vi "Asylum_Driver_Plugin_IVCurve.vi"(4 "Abort Notifier":refnum<notifier>, 6 "Interpolation":dbl format="%#_13g", 7 "Writing Setpoint":dbl=0.1 format="%#_13g", 8 "error in (no error)":errorcluster, 9 "Offsets":cluster{"X":dbl, "Y":dbl}, 10 "Pattern Data":T2={"Name"="", "Litho"=[], "Set Resistance"=enum."1G ohm", "Meta"=variant}, 11 "Application":refnum<k7>) -> (0 "error out":errorcluster, 1 "Y":dbl[](array[numeric]), 2 "X":dbl[](array[numeric]), 3 "Application Out":refnum<k7>)   [LabVIEW 2019]
uses:
  <userlib>/LevyLab/RemoteControl/RemoteControl/RemoteControl.lvclass
  <userlib>/LevyLab/Instrument Framework/SMOs/RemoteControl/RemoteControl.lvclass
  Classes/Settings/Dot Settings/TypeDefs/IV Settings.ctl
  Classes/Settings/Dot Settings/Dot Settings.lvclass
  <userlib>/LevyLab/RemoteControl/RemoteControl/Typedefs/RC Com Type--enum.ctl
  0e2d323c-3e35-47fb-9129-4c7af1e32b05.vi
  43673bb9-479d-403d-a5d0-439c933431c4.vi
  a6f932bf-8dea-4ae5-a866-4f706d76ef40.vi
  7c826ca2-1f29-4c4d-bf7c-0946160d1343.vi
  0945bc12-bc18-4d8f-896b-f5f56bd4a894.vi
  3a94caf1-4aca-4e02-84db-939cfa50ca80.vi
  <userlib>/LevyLab/Relay Box/Typedefs/Resistor--enum.ctl
  <userlib>/LevyLab/Relay Box/Relay-Box.lvclass
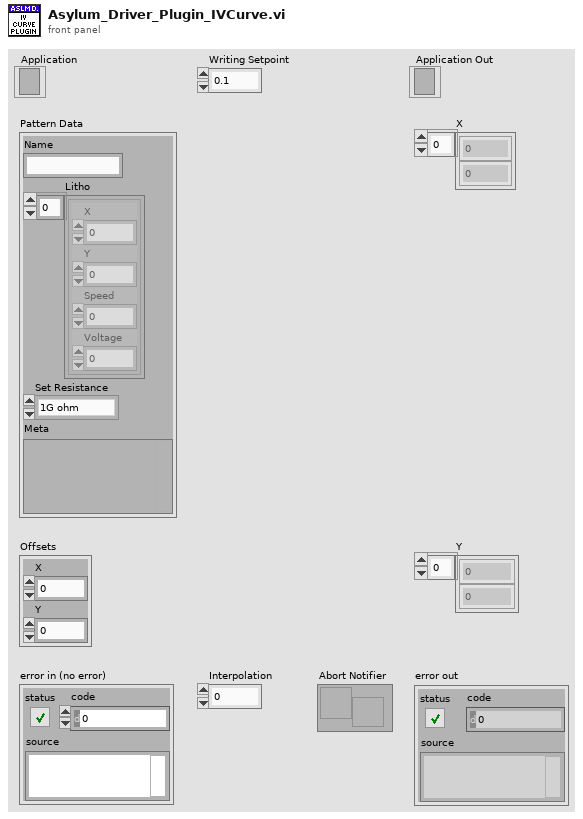
[diagram p1: front panel]
types:
  T1 = typedef "Relay-Box.lvclass/Resistor--enum.ctl" = enum16{"open", "discharge tip", "0 ohms", "100k ohm", "10M ohm", "1G ohm"}
  T2 = cluster{"Name":string, "Litho":cluster{"X":dbl, "Y":dbl, "Speed":dbl, "Voltage":dbl}[], "Set Resistance":T1, "Meta":variant}
  T3 = enum32{"Invalid", "Standard", "Closed", "Hidden", "Minimized", "Maximized"}
  T4 = enum32{"invalid app kind", "Development System", "Run Time System", "Student Edition", "Embedded LabVIEW", "Evaluation", "Custom"}
  T5 = typedef "RemoteControl.lvlib/RemoteControl.lvclass/RC Com Type--enum.ctl" = enum16{"RC", "STM", "ZMQ"}
  T6 = cluster{"Pattern":enum16{"Ramp /", "Ramp /\\", "Smooth Ramp _/", "Smooth Ramp _/\\_", "Frequency"}, "Cycles":i32, "Rate":dbl, "End":dbl, "Start":dbl}
  T7 = enum16{"Ramp /", "Ramp /\\", "Smooth Ramp _/", "Smooth Ramp _/\\_", "Frequency"}
  T8 = typedef "Dot Settings.lvclass/IV Settings.ctl" = cluster{"Pattern":enum16{"Ramp /", "Ramp /\\", "Smooth Ramp _/", "Smooth Ramp _/\\_", "Frequency"}, "Cycles":i32, "Rate":dbl, "End":dbl, "Start":dbl, "Port":u32, "Time":dbl, "Points":dbl[]}
  T9 = cluster{"Core":cluster{"Current VI Reference":refnum<vi>, "Close Panel on Exit?":bool}, "Application":refnum<k7>, "Writing Setpoint":dbl, "Offsets":cluster{"X":dbl, "Y":dbl}, "Interpolation":dbl, "Pattern Data":cluster{"Name":string, "Litho":cluster{"X":dbl, "Y":dbl, "Speed":dbl, "Voltage":dbl}[], "Set Resistance":T1, "Meta":variant}, "Abort Notifier":refnum<notifier>, "RemoteControl":refnum<class "RemoteControl.lvclass">, "IV Settings":T8, "Status":enum16{"IDLE", "RUNNING", "FINISHED", "ABORTED"}, "Timeout":u32, "Plugin Status":i32}
  T10 = cluster{"Current VI Reference":refnum<vi>, "Close Panel on Exit?":bool}
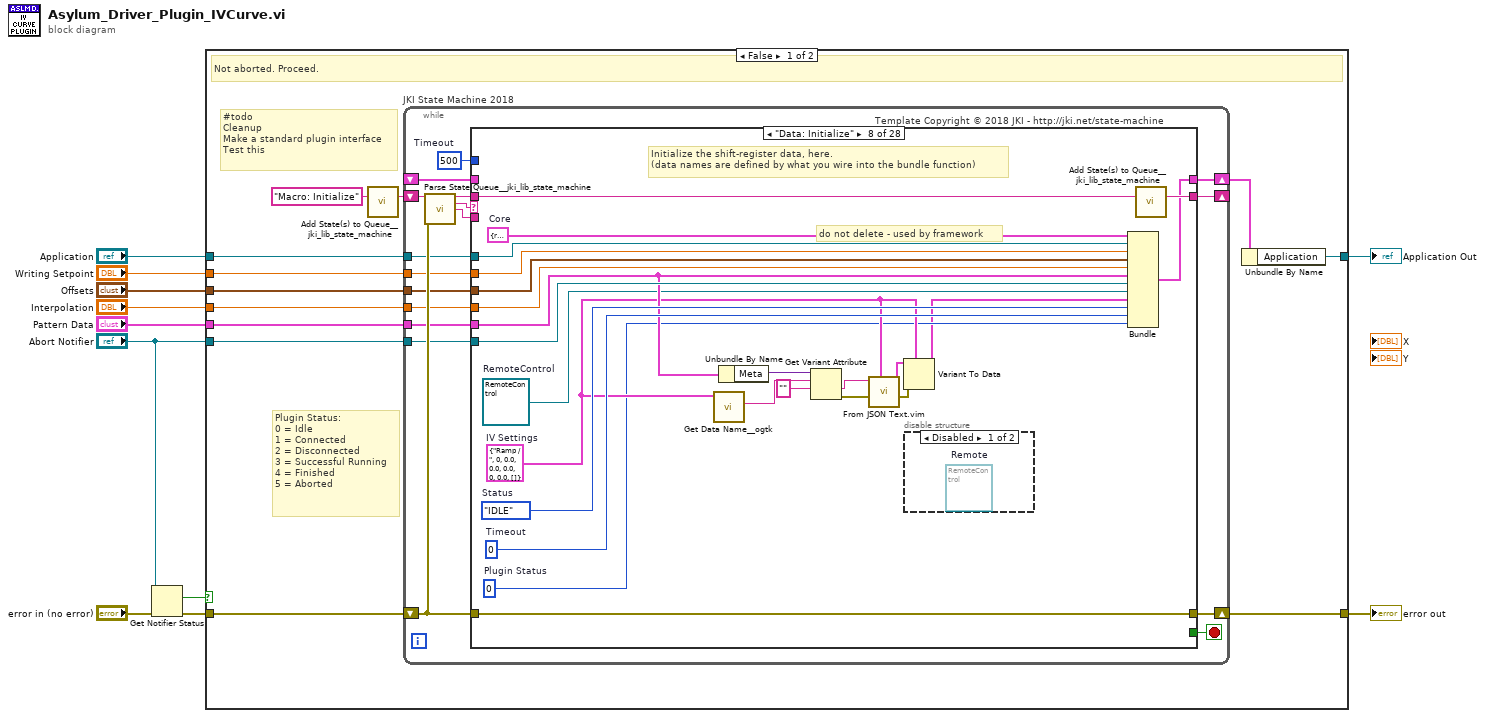
[diagram p0: block diagram]
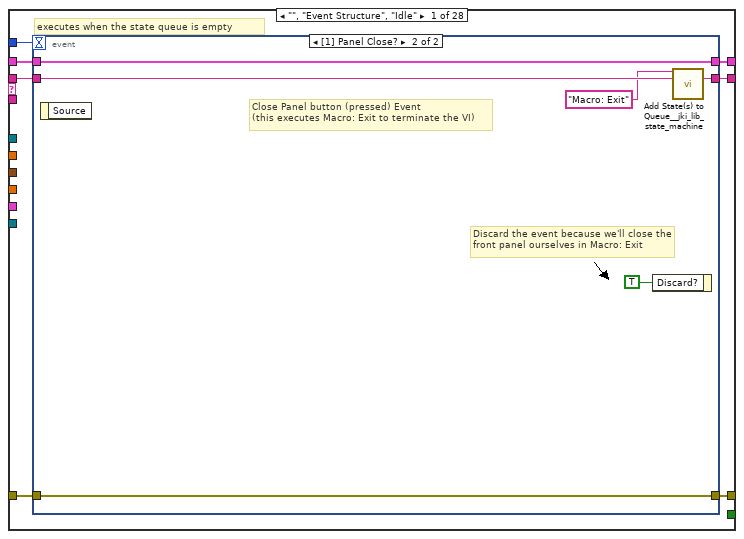
[diagram p2: hidden frame]
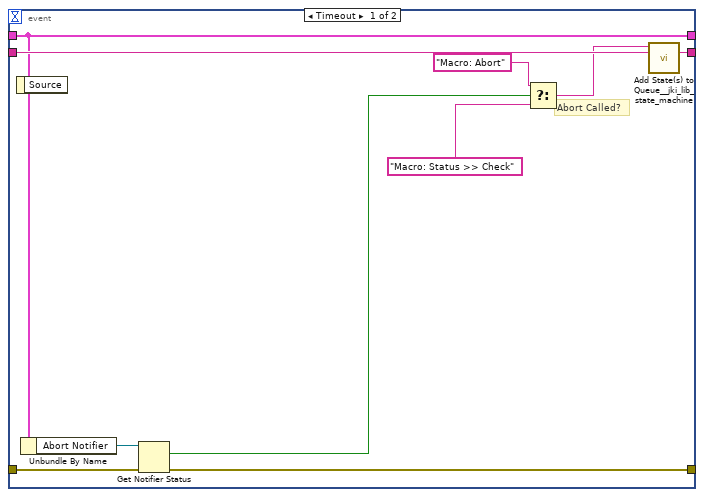
[diagram p3: hidden frame]
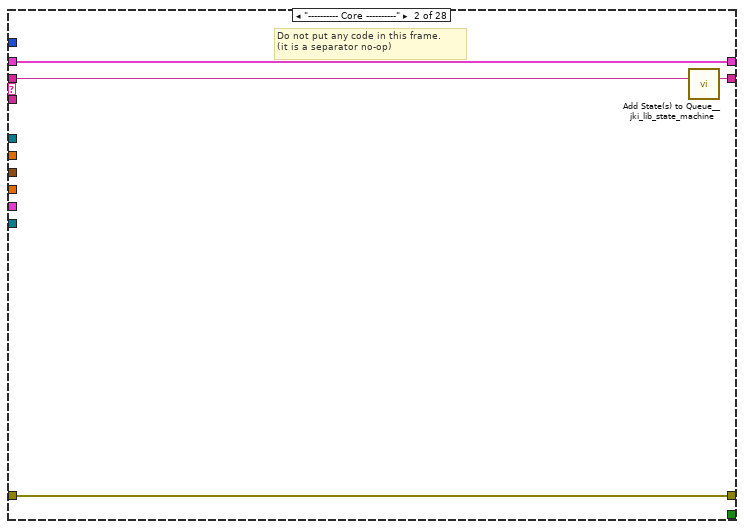
[diagram p4: hidden frame]
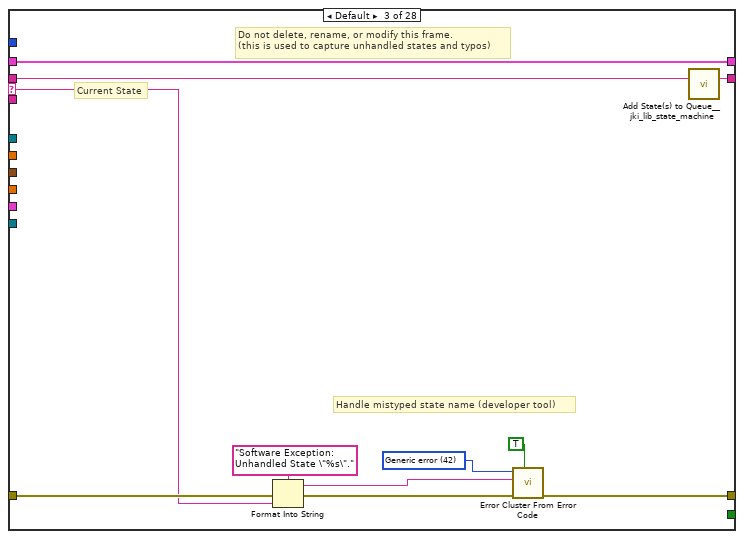
[diagram p5: hidden frame]
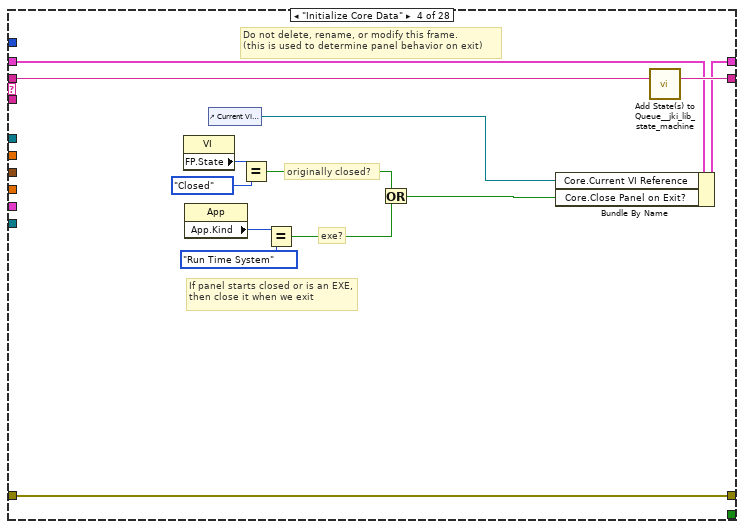
[diagram p6: hidden frame]
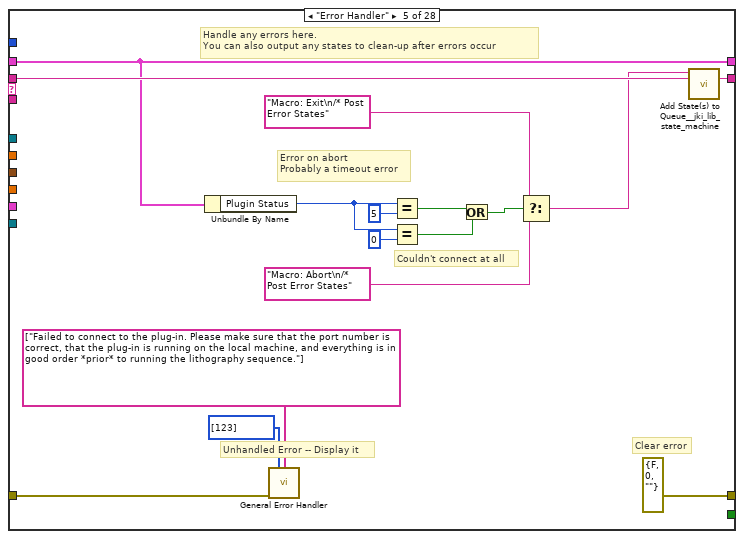
[diagram p7: hidden frame]
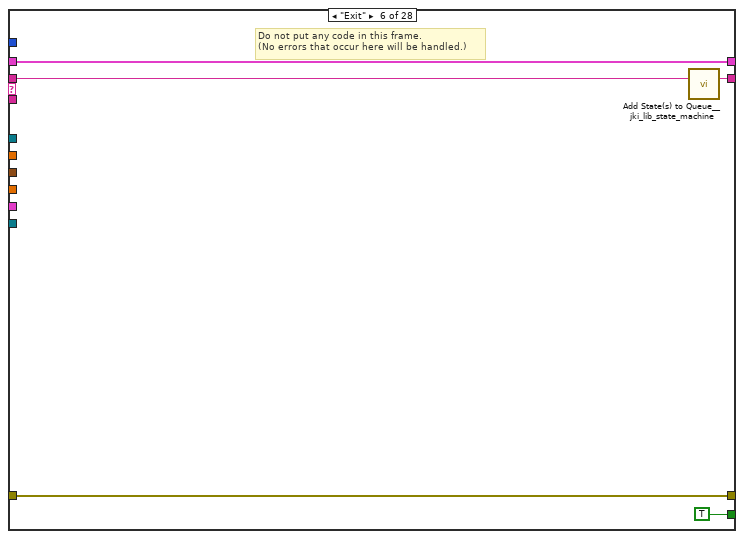
[diagram p8: hidden frame]
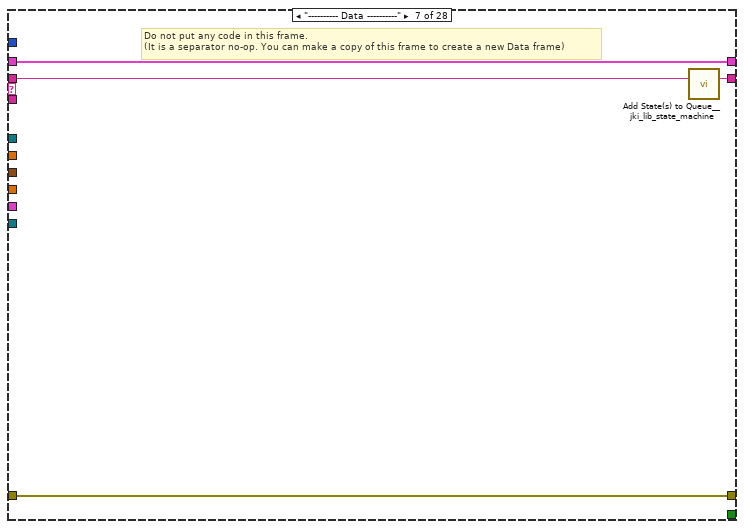
[diagram p9: hidden frame]
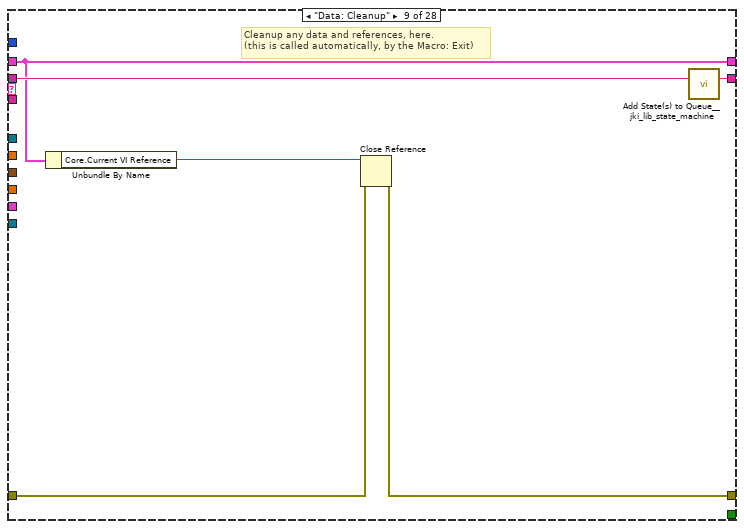
[diagram p11: hidden frame]
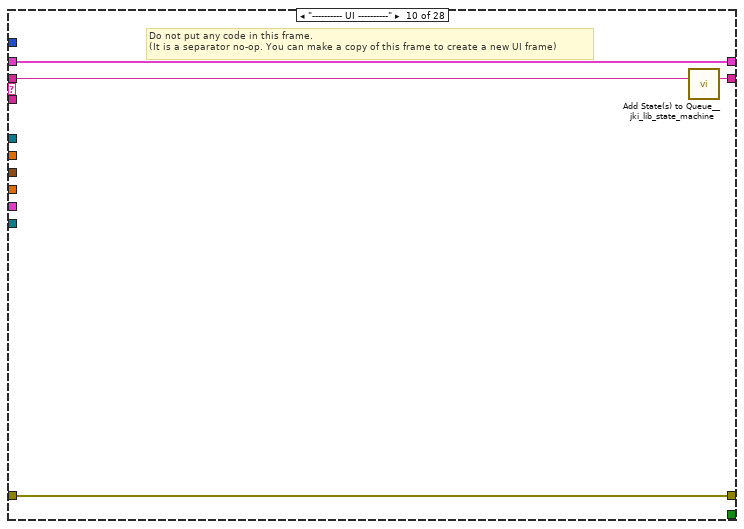
[diagram p12: hidden frame]
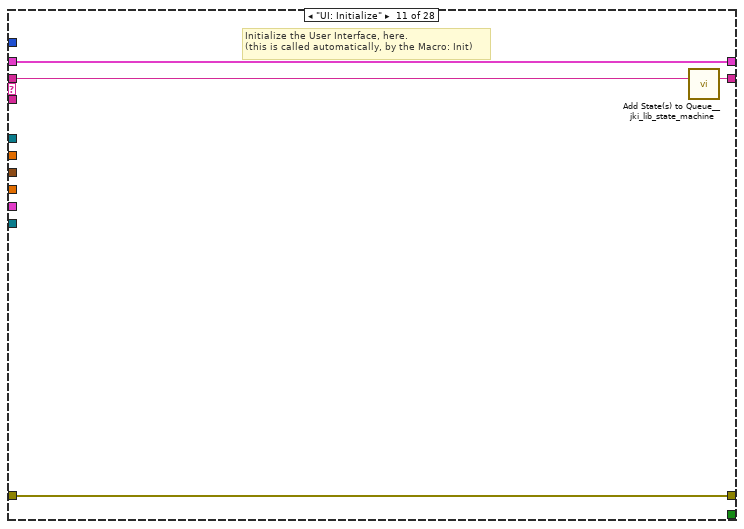
[diagram p13: hidden frame]
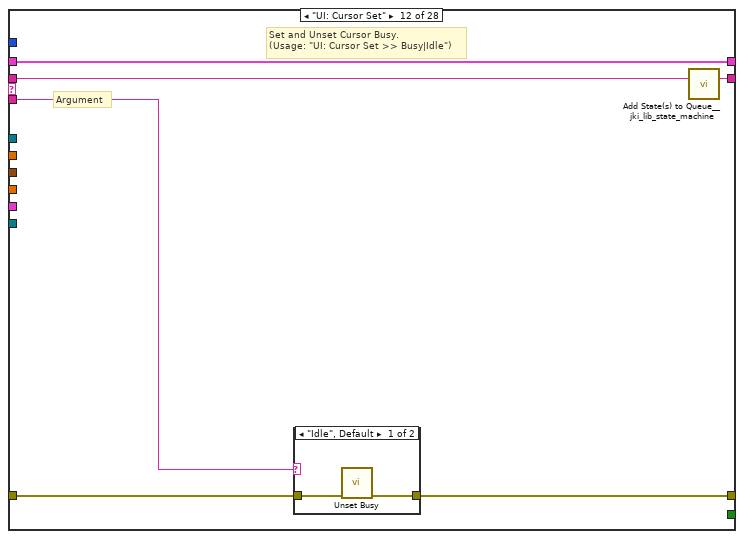
[diagram p14: hidden frame]
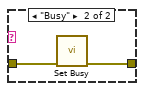
[diagram p15: hidden frame]
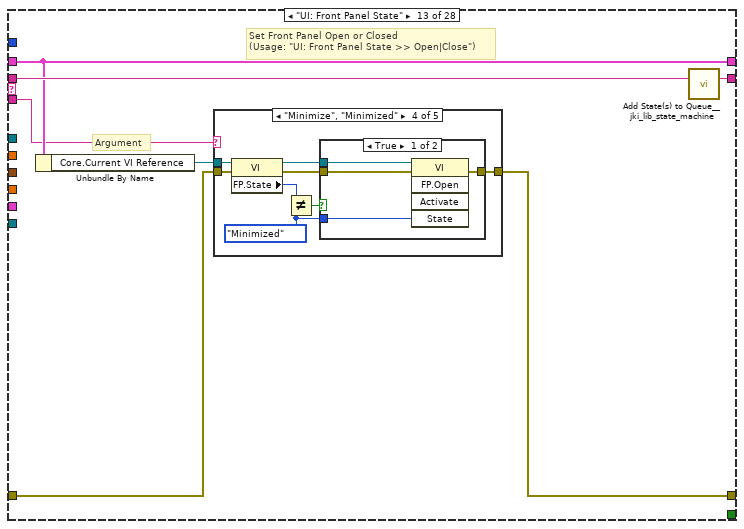
[diagram p16: hidden frame]
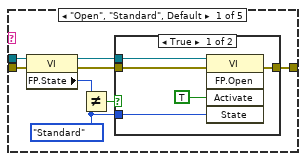
[diagram p17: hidden frame]
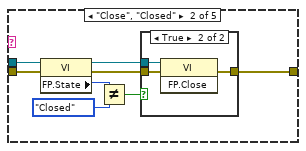
[diagram p19: hidden frame]
diagram:
  n1 = Get Notifier Status(notifier="Abort Notifier", error in (no error)="error in (no error)") -> (current notification=w1:bool, error out=w3:errorcluster)  [unwired: 3 out]
  n2 = case shown="False" w1 {
    tunnel: [w21 w451] -> w11
    tunnel: "Application" -> [w20 w452]
    tunnel: "Writing Setpoint" -> [w19 _]
    tunnel: "Offsets" -> [w18 _]
    tunnel: "Interpolation" -> [w17 _]
    tunnel: "Pattern Data" -> [w16 _]
    tunnel: [w15 w452] -> w5
    tunnel: w3 -> [w14 w451]
    tunnel: "Abort Notifier" -> [w13 _]
    frame False {
      # "Plugin Status:\n0 = Idle\n1 = Connected\n2 = Disconnected\n3 = Successful Running\n4 = Finished\n5 = Aborted"
      # "#todo\nCleanup\nMake a standard plugin interface\nTest this"
      # "Not aborted. Proceed."
      n3 = call <vilib>:"Add State(s) to Queue__jki_lib_state_machine.vi"("State(s) in (\"\")"="Macro: Initialize") -> ("States Out"=w23:string)  [unwired: 14 in]
      n4 = while "JKI State Machine 2018" {
        shift-right: [w33] -> w12
        shift-left: _ -> [w32]
        shift-right: [w36] -> w21
        shift-left: w14 -> [w30]
        shift-right: [w35] -> _
        shift-left: w23 -> [w37]
        tunnel: w20 -> [w29]
        tunnel: w19 -> [w28]
        tunnel: w18 -> [w27]
        tunnel: w17 -> [w26]
        tunnel: w16 -> [w25]
        tunnel: w13 -> [w24]
        stop <- w34 stop-if-true
        w31 = 500  # Timeout
        # "Template Copyright © 2018 JKI - http://jki.net/state-machine"
        n5 = call <vilib>:"Parse State Queue__jki_lib_state_machine.vi"("State Queue"=w37, "Error In (no error)"=w30) -> ("Remaining States"=w39:string, "Current State"=w40:string, "Arguments"=w38:string)  [unwired: 11 in]
        n6 = case shown="\"Data: Initialize\"" w40 {
          selector: w40 -> [_ _ w68 _ _ _ _ _ _ _ _ _ _ _ _ _ _ _ _ _ _ _ _ _ _ _ _ _]
          tunnel: w39 -> [w47 w67 w72 w91 w107 w112 w116 w140 w146 w150 w154 w160 w171 w240 w247 w260 w265 w275 w287 w305 w316 w333 w365 w384 w388 w398 w408 w414]
          tunnel: w38 -> [_ _ _ _ _ _ _ _ _ _ _ w155 w165 _ w244 _ _ _ _ _ _ _ _ _ _ _ _ _]
          tunnel: w32 -> [w45 w64 w70 w84 w104 w110 w113 _ w141 w147 w152 w158 w167 w237 w243 w257 w262 w272 w282 w302 w313 w328 w360 w379 w385 w395 w405 w410]
          tunnel: [w44 w65 w74 w88 errorcluster {"status"=FALSE, "code"=0, "source"=""} ("error out") w109 w114 w137 w142 w148 w151 w156 w168 w238 w245 w258 w263 w273 w278 w289 w306 w319 w347 w371 w386 w391 w406 w412] -> w36
          tunnel: w30 -> [w43 w65 w73 w88 w94 w109 w114 w137 w143 w148 w151 w157 w169 w238 w245 w258 w263 w273 w281 w300 w310 w318 w338 w366 w386 w390 w406 w412]
          tunnel: [w46 w66 w71 w90 w106 w111 w115 w139 w145 w149 w153 w159 w170 w239 w246 w259 w264 w274 w286 w304 w315 w332 w364 w383 w387 w397 w407 w413] -> w35
          tunnel: [_ _ _ _ _ TRUE _ _ _ _ _ _ _ _ _ _ _ _ _ _ _ _ _ _ _ _ _ _] -> w34
          tunnel: [w42 w64 w70 w89 w104 w110 w113 w138 w141 w147 w152 w158 w167 w237 w243 w257 w262 w272 w283 w303 w314 w329 w361 w380 w385 w395 w405 w411] -> w33
          tunnel: w31 -> [w41 _ _ _ _ _ _ _ _ _ _ _ _ _ _ _ _ _ _ _ _ _ _ _ _ _ _ _]
          tunnel: w29 -> [_ _ _ _ _ _ _ w135 _ _ _ _ _ _ _ _ _ _ _ _ _ _ _ _ _ _ _ _]
          tunnel: w28 -> [_ _ _ _ _ _ _ w134 _ _ _ _ _ _ _ _ _ _ _ _ _ _ _ _ _ _ _ _]
          tunnel: w27 -> [_ _ _ _ _ _ _ w133 _ _ _ _ _ _ _ _ _ _ _ _ _ _ _ _ _ _ _ _]
          tunnel: w26 -> [_ _ _ _ _ _ _ w132 _ _ _ _ _ _ _ _ _ _ _ _ _ _ _ _ _ _ _ _]
          tunnel: w25 -> [_ _ _ _ _ _ _ w128 _ _ _ _ _ _ _ _ _ _ _ _ _ _ _ _ _ _ _ _]
          tunnel: w24 -> [_ _ _ _ _ _ _ w131 _ _ _ _ _ _ _ _ _ _ _ _ _ _ _ _ _ _ _ _]
          frame "", "Event Structure", "Idle" {
            # "executes when the state queue is empty"
            n7 = event shown="[1] Panel Close?" {
              selector: _ -> [_ _]
              dyn-events: _ -> [_ _]
              timeout: w41 -> [_ _]
              tunnel: w47 -> [w57 w63]
              tunnel: [w56 w62] -> w46
              tunnel: w45 -> [w55 w60]
              tunnel: [w54 w61] -> w44
              tunnel: w43 -> [w53 w61]
              tunnel: [w55 w60] -> w42
              event Timeout {
                # "Abort Called?"
                n8 = event-data() -> ()  [unwired: 1 in, 1 out]
                n9 = Unbundle By Name(w55) -> ("Abort Notifier"=w52:refnum<notifier>)
                n10 = Get Notifier Status(notifier=w52, error in (no error)=w53) -> (current notification=w48:bool, error out=w54:errorcluster)  [unwired: 3 out]
                n11 = Select(t="Macro: Abort", s=w48, f="Macro: Status >> Check" ("t")) -> (s? t:f=w51:string)
                n12 = call <vilib>:"Add State(s) to Queue__jki_lib_state_machine.vi"("State(s) in Front (\"\")"=w51, "State(s) in (\"\")"=w57) -> ("States Out"=w56:string)  [unwired: 13 in]
              }
              event Panel Close? {
                # "Discard the event because we'll close the front panel ourselves in Macro: Exit"
                # "Close Panel button (pressed) Event\n(this executes Macro: Exit to terminate the VI)"
                n13 = event-data() -> ()  [unwired: 1 in, 1 out]
                n14 = event-data("Discard?"=TRUE) -> ()  [unwired: 1 in, 1 out]
                n15 = call <vilib>:"Add State(s) to Queue__jki_lib_state_machine.vi"("State(s) in Front (\"\")"="Macro: Exit", "State(s) in (\"\")"=w63) -> ("States Out"=w62:string)  [unwired: 13 in]
              }
            }
          }
          frame "---------- Core ----------" {
            # "Do not put any code in this frame.\n(it is a separator no-op)"
            n16 = call <vilib>:"Add State(s) to Queue__jki_lib_state_machine.vi"("State(s) in (\"\")"=w67) -> ("States Out"=w66:string)  [unwired: 14 in]
          }
          frame Default {
            w77 = 42 items=["No error", "Argument error", "Memory is full", "Out of zone", "End of file", "File already open", "Generic file I/O error", "File not found", "File permission error", "Disk is full", "Duplicate path", "Too many files open", "System feature not enabled", "Resource file not found", "Cannot add resource", "Resource not found", "Image not found", "Image memory error", "Pen does not exist", "Config type invalid", "Config token not found", "Config parse error", "Config memory error", "Bad external code format", "Bad external code offset", "External code not present", "Null window", "Destroy window error", "Null menu", "Print aborted", "Bad print record", "Print driver error", "Windows error during printing", "Memory error during printing", "Print dialog error", "Generic print error", "Invalid device refnum", "Device not found", "Device parameter error", "Device unit error", "Cannot open device", "Device call aborted", "Generic error", "Cancelled by user", "Object ID too low", "Object ID too high", "Object not in heap", "Unknown heap", "Unknown object (invalid DefProc)", "Unknown object (DefProc not in table)", "Message out of range", "Invalid (null) method", "Unknown message", "Manager call not supported", "Bad address", "Network operation in progress", "Network operation timed out", "Connection is busy", "Network attribute not supported", "Network error", "Address in use", "System out of memory", "Connection aborted", "Connection refused", "Not connected", "Already connected", "Connection closed", "Initialization error (interapplication manager)", "Bad occurrence", "Wait on unbound occurrence handler", "Occurrence queue overflow", "Datalog type conflict", "Unused", "Unrecognized type (interapplication manager)", "Memory corrupt", "Failed to make temporary DLL", "Old CIN version", "Drag socket not found", "Failed to load drop-object", "Failed to register OLE object", "Failed to release OLE object", "Format specifier type mismatch", "Unknown format specifier", "Too few format specifiers", "Too many format specifiers", "Scan failed", "Newer CIN version", "Error converting to variant", "Runtime menu error", "Password tampered", "Variant attribute not found", "Incompatible variant data type", "Event data is not available", "Event Store is not present", "Occurrence is not found", "Event Queue is not created", "Event info is not available", "Refnum passed is NULL", "Error retrieving Class GUID", "Error retrieving CoClass GUID", "Error retrieving TypeLib GUID.", "Bad built application magic bytes.", "Specific driver is different from the specific driver associated with the Logical Name.", "There is no session opened to the class driver.", "Max Error", "MAX - Error with config objects", "MAX - Error loading configuration", "MAX - Group not supported"]
            # "Current State"
            # "Do not delete, rename, or modify this frame.\n(this is used to capture unhandled states and typos)"
            # "Handle mistyped state name (developer tool)"
            n17 = Format Into String(format string="Software Exception: Unhandled State \"%s\"." ("message"), error in=w73, w68) -> (resulting string=w76:string, error out=w75:errorcluster)  [unwired: 1 in]
            n18 = call <vilib>:"Error Cluster From Error Code.vi"("show call chain? (False)"=TRUE, "error in (no error)"=w75, "error message (\"\")"=w76, "error code (0)"=w77) -> ("error out"=w74:errorcluster)  [unwired: 5 in]
            n19 = call <vilib>:"Add State(s) to Queue__jki_lib_state_machine.vi"("State(s) in (\"\")"=w72) -> ("States Out"=w71:string)  [unwired: 14 in]
          }
          frame "Initialize Core Data" {
            # "Do not delete, rename, or modify this frame.\n(this is used to determine panel behavior on exit)"
            # "originally closed?"
            # "exe?"
            # "If panel starts closed or is an EXE, then close it when we exit"
            n20 = property class="VI"() -> ("FP.State"=w81:T3)  [unwired: 2 in, 2 out]
            n21 = property class="App"() -> ("App.Kind"=w87:T4)  [unwired: 2 in, 2 out]
            n22 = control-ref of="Current VI Reference"() -> (w82:refnum<vi>)
            n23 = Equal?(x=w81, y=T3."Closed" ("Front Panel Window:State")) -> (x = y?=w79:bool)
            n24 = Equal?(x=w87, y=T4."Run Time System" ("Application:Kind")) -> (x = y?=w85:bool)
            n25 = Or(x=w79, y=w85) -> (x .or. y?=w83:bool)
            n26 = Bundle By Name(cluster=w84, "Core.Current VI Reference"=w82, "Core.Close Panel on Exit?"=w83) -> (w89:T9)
            n27 = call <vilib>:"Add State(s) to Queue__jki_lib_state_machine.vi"("State(s) in (\"\")"=w91) -> ("States Out"=w90:string)  [unwired: 14 in]
          }
          frame "Error Handler" {
            # "Couldn't connect at all"
            # "Error on abort\nProbably a timeout error"
            # "Unhandled Error -- Display it"
            # "Handle any errors here.\nYou can also output any states to clean-up after errors occur"
            # "Clear error"
            n28 = Unbundle By Name(w104) -> ("Plugin Status"=w97:i32)
            n29 = call <vilib>:"General Error Handler.vi"("[user-defined codes]"=i32[] [123], "[user-defined descriptions]"=string[] ["Failed to connect to the plug-in. Please make sure that the port number is correct, that the plug-in is running on the local machine, and everything is in good order *prior* to running the lithography sequence."], "error in (no error)"=w94) -> ()  [unwired: 8 in, 5 out]
            n30 = Equal?(x=w97, y=5) -> (x = y?=w99:bool)
            n31 = Equal?(x=w97, y=0) -> (x = y?=w95:bool)
            n32 = Or(x=w99, y=w95) -> (x .or. y?=w98:bool)
            n33 = Select(t="Macro: Exit\n/* Post Error States", s=w98, f="Macro: Abort\n/* Post Error States") -> (s? t:f=w100:string)
            n34 = call <vilib>:"Add State(s) to Queue__jki_lib_state_machine.vi"("State(s) in Front (\"\")"=w100, "State(s) in (\"\")"=w107) -> ("States Out"=w106:string)  [unwired: 13 in]
          }
          frame "Exit" {
            # "Do not put any code in this frame.\n(No errors that occur here will be handled.)"
            n35 = call <vilib>:"Add State(s) to Queue__jki_lib_state_machine.vi"("State(s) in (\"\")"=w112) -> ("States Out"=w111:string)  [unwired: 14 in]
          }
          frame "---------- Data ----------" {
            # "Do not put any code in this frame.\n(It is a separator no-op. You can make a copy of this frame to create a new Data frame)"
            n36 = call <vilib>:"Add State(s) to Queue__jki_lib_state_machine.vi"("State(s) in (\"\")"=w116) -> ("States Out"=w115:string)  [unwired: 14 in]
          }
          frame "Data: Initialize" {
            w117 = refnum<class "RemoteControl.lvclass"> refnum  # RemoteControl
            w119 = 0  # Plugin Status
            w129 = u32 0  # Timeout
            w130 = enum16{"IDLE", "RUNNING", "FINISHED", "ABORTED"}."IDLE"  # Status
            w122 = T8 {"Pattern"=enum."Ramp /", "Cycles"=0, "Rate"=0.0, "End"=0.0, "Start"=0.0, "Port"=0, "Time"=0.0, "Points"=[]}  # IV Settings
            w136 = T10 {"Current VI Reference"=refnum, "Close Panel on Exit?"=FALSE}  # Core
            # "do not delete - used by framework"
            # "Initialize the shift-register data, here.\n(data names are defined by what you wire into the bundle function)"
            n37 = call <userlib>:"Get Data Name__ogtk.vi"("Data"=w122) -> ("Data Name"=w126:string)  [unwired: 8 in, 2 out]
            n38 = Unbundle By Name(w128) -> ("Meta"=w127:variant)
            n39 = Get Variant Attribute(Variant=w127, name=w126, default value (empty Variant)="") -> (value=w121:string, error out=w124:errorcluster)  [unwired: 1 in, 2 out]
            n40 = call "From JSON Text.vim"("Data Type and Default Value"=w122, "error in (no error)"=w124, "JSON"=w121) -> ("error out"=w123:errorcluster, "Data out"=w120:T8)  [unwired: 7 in]
            n41 = Variant To Data(error in=w123, type=w122, Variant=w120) -> (data=w118:T8)  [unwired: 1 out]
            n42 = disable-structure shown="Disabled" {
              frame Disabled {
                (unwired) refnum<class "RemoteControl.lvclass"> refnum  # Remote
              }
              frame Enabled {
              }
            }
            n43 = Bundle("Core"=w136, "Application"=w135, "Writing Setpoint"=w134, "Offsets"=w133, "Interpolation"=w132, "Pattern Data"=w128, "Abort Notifier"=w131, "RemoteControl"=w117, "IV Settings"=w118, "Status"=w130, "Timeout"=w129, "Plugin Status"=w119) -> (w138:T9)  [unwired: 1 in]
            n44 = call <vilib>:"Add State(s) to Queue__jki_lib_state_machine.vi"("State(s) in (\"\")"=w140) -> ("States Out"=w139:string)  [unwired: 14 in]
          }
          frame "Data: Cleanup" {
            # "Cleanup any data and references, here.\n(this is called automatically, by the Macro: Exit)"
            n45 = Unbundle By Name(w141) -> ("Core.Current VI Reference"=w144:refnum<vi>)
            n46 = Close Reference(reference=w144, error in (no error)=w143) -> (error out=w142:errorcluster)
            n47 = call <vilib>:"Add State(s) to Queue__jki_lib_state_machine.vi"("State(s) in (\"\")"=w146) -> ("States Out"=w145:string)  [unwired: 14 in]
          }
          frame "---------- UI ----------" {
            # "Do not put any code in this frame.\n(It is a separator no-op. You can make a copy of this frame to create a new UI frame)"
            n48 = call <vilib>:"Add State(s) to Queue__jki_lib_state_machine.vi"("State(s) in (\"\")"=w150) -> ("States Out"=w149:string)  [unwired: 14 in]
          }
          frame "UI: Initialize" {
            # "Initialize the User Interface, here.\n(this is called automatically, by the Macro: Init)"
            n49 = call <vilib>:"Add State(s) to Queue__jki_lib_state_machine.vi"("State(s) in (\"\")"=w154) -> ("States Out"=w153:string)  [unwired: 14 in]
          }
          frame "UI: Cursor Set" {
            # "Argument"
            # "Set and Unset Cursor Busy.\n(Usage: \"UI: Cursor Set >> Busy|Idle\")"
            n50 = case shown="\"Idle\", Default" w155 {
              tunnel: w157 -> [w162 w164]
              tunnel: [w161 w163] -> w156
              frame "Idle", Default {
                n51 = call <vilib>:"Unset Busy.vi"("error in (no error)"=w162) -> ("error out"=w161:errorcluster)  [unwired: 10 in]
              }
              frame "Busy" {
                n52 = call <vilib>:"Set Busy.vi"("error in (no error)"=w164) -> ("error out"=w163:errorcluster)  [unwired: 9 in, 1 out]
              }
            }
            n53 = call <vilib>:"Add State(s) to Queue__jki_lib_state_machine.vi"("State(s) in (\"\")"=w160) -> ("States Out"=w159:string)  [unwired: 14 in]
          }
          frame "UI: Front Panel State" {
            # "Argument"
            # "Set Front Panel Open or Closed\n(Usage: \"UI: Front Panel State >> Open|Close\")"
            n54 = Unbundle By Name(w167) -> ("Core.Current VI Reference"=w166:refnum<vi>)
            n55 = case shown="\"Minimize\", \"Minimized\"" w165 {
              tunnel: w169 -> [w177 w192 w203 w216 w229]
              tunnel: [w179 w193 w205 w218 w231] -> w168
              tunnel: w166 -> [w178 w190 w204 w217 w230]
              frame "Open", "Standard", Default {
                w172 = T3."Standard" ("State")
                n56 = property class="VI"(reference=w178, error in=w177) -> (reference out=w175:refnum<vi>, error out=w176:errorcluster, "FP.State"=w174:T3)
                n57 = Not Equal?(x=w174, y=w172) -> (x != y?=w173:bool)
                n58 = case shown="True" w173 {
                  tunnel: [w183 w185] -> w179
                  tunnel: w176 -> [w182 w185]
                  tunnel: w175 -> [w181 _]
                  tunnel: w172 -> [w180 _]
                  frame True {
                    n59 = invoke class="VI" method="FP.Open"(reference=w181, error in=w182, "Activate"=TRUE, "State"=w180) -> (error out=w183:errorcluster)  [unwired: 1 in, 4 out]
                  }
                  frame False {
                  }
                }
              }
              frame "Close", "Closed" {
                n60 = property class="VI"(reference=w190, error in=w192) -> (reference out=w189:refnum<vi>, error out=w191:errorcluster, "FP.State"=w187:T3)
                n61 = Not Equal?(x=w187, y=T3."Closed" ("Front Panel Window:State")) -> (x != y?=w186:bool)
                n62 = case shown="True" w186 {
                  tunnel: [w194 w197] -> w193
                  tunnel: w191 -> [w194 w196]
                  tunnel: w189 -> [_ w195]
                  frame False {
                  }
                  frame True {
                    n63 = invoke class="VI" method="FP.Close"(reference=w195, error in=w196) -> (error out=w197:errorcluster)  [unwired: 1 in, 2 out]
                  }
                }
              }
              frame "Hidden", "Hide" {
                w198 = T3."Hidden" ("State")
                n64 = property class="VI"(reference=w204, error in=w203) -> (reference out=w201:refnum<vi>, error out=w202:errorcluster, "FP.State"=w200:T3)
                n65 = Not Equal?(x=w200, y=w198) -> (x != y?=w199:bool)
                n66 = case shown="True" w199 {
                  tunnel: [w209 w210] -> w205
                  tunnel: w202 -> [w208 w210]
                  tunnel: w201 -> [w207 _]
                  tunnel: w198 -> [w206 _]
                  frame True {
                    n67 = invoke class="VI" method="FP.Open"(reference=w207, error in=w208, "State"=w206) -> (error out=w209:errorcluster)  [unwired: 2 in, 4 out]
                  }
                  frame False {
                  }
                }
              }
              frame "Minimize", "Minimized" {
                w211 = T3."Minimized" ("State")
                n68 = property class="VI"(reference=w217, error in=w216) -> (reference out=w214:refnum<vi>, error out=w215:errorcluster, "FP.State"=w213:T3)
                n69 = Not Equal?(x=w213, y=w211) -> (x != y?=w212:bool)
                n70 = case shown="True" w212 {
                  tunnel: [w222 w223] -> w218
                  tunnel: w215 -> [w221 w223]
                  tunnel: w214 -> [w220 _]
                  tunnel: w211 -> [w219 _]
                  frame True {
                    n71 = invoke class="VI" method="FP.Open"(reference=w220, error in=w221, "State"=w219) -> (error out=w222:errorcluster)  [unwired: 2 in, 4 out]
                  }
                  frame False {
                  }
                }
              }
              frame "Maximize", "Maximized" {
                w224 = T3."Maximized" ("State")
                n72 = property class="VI"(reference=w230, error in=w229) -> (reference out=w227:refnum<vi>, error out=w228:errorcluster, "FP.State"=w226:T3)
                n73 = Not Equal?(x=w226, y=w224) -> (x != y?=w225:bool)
                n74 = case shown="True" w225 {
                  tunnel: [w235 w236] -> w231
                  tunnel: w228 -> [w234 w236]
                  tunnel: w227 -> [w233 _]
                  tunnel: w224 -> [w232 _]
                  frame True {
                    n75 = invoke class="VI" method="FP.Open"(reference=w233, error in=w234, "State"=w232) -> (error out=w235:errorcluster)  [unwired: 2 in, 4 out]
                  }
                  frame False {
                  }
                }
              }
            }
            n76 = call <vilib>:"Add State(s) to Queue__jki_lib_state_machine.vi"("State(s) in (\"\")"=w171) -> ("States Out"=w170:string)  [unwired: 14 in]
          }
          frame "---------- Macro ----------" {
            # "Do not put any code in this frame.\n(It is a separator no-op. You can make a copy of this frame to create a new Macro frame)"
            n77 = call <vilib>:"Add State(s) to Queue__jki_lib_state_machine.vi"("State(s) in (\"\")"=w240) -> ("States Out"=w239:string)  [unwired: 14 in]
          }
          frame "Macro: Status" {
            # "Do not put any code in this frame.\n(It is a separator no-op. You can make a copy of this frame to create a new Macro frame)"
            n78 = Unbundle By Name(w243) -> ("Status"=w242:enum16{"IDLE", "RUNNING", "FINISHED", "ABORTED"})
            n79 = case shown="\"Interpret\"" w244 {
              tunnel: w242 -> [_ _ w251]
              tunnel: ["Default" "Remote: IV_STATUS\nMacro: Status >> Interpret" w250] -> w241
              frame Default {
              }
              frame "Check" {
              }
              frame "Interpret" {
                n80 = case shown="\"IDLE\", \"RUNNING\"" w251 {
                  tunnel: ["" "Macro: Exit" "Macro: Exit" "Timeout: Check"] -> w250
                  frame Default {
                  }
                  frame "ABORTED" {
                  }
                  frame "FINISHED" {
                  }
                  frame "IDLE", "RUNNING" {
                  }
                }
              }
            }
            n81 = call <vilib>:"Add State(s) to Queue__jki_lib_state_machine.vi"("State(s) in Front (\"\")"=w241, "State(s) in (\"\")"=w247) -> ("States Out"=w246:string)  [unwired: 13 in]
          }
          frame "Macro: Abort" {
            # "Do not put any code in this frame.\n(It is a separator no-op. You can make a copy of this frame to create a new Macro frame)"
            n82 = call <vilib>:"Add State(s) to Queue__jki_lib_state_machine.vi"("State(s) in Front (\"\")"="Remote: IV_ABORT\nMacro: Exit", "State(s) in (\"\")"=w260) -> ("States Out"=w259:string)  [unwired: 13 in]
          }
          frame "Macro: Initialize" {
            w261 = "Data: Initialize\nInitialize Core Data\n//UI: Initialize\n//UI: Front Panel State >> Open\nRemote: Connect\nRemote: IV_RUN\nTimeout: Calculate"  # Data: Initialize Initialize Core Data //UI: Initialize //UI: Front Panel State >> Open Remote: Connect Remote: IV_RUN Timeout: Calculate
            # "Initialization Macro\n(This is called once, when the VI starts)"
            n83 = call <vilib>:"Add State(s) to Queue__jki_lib_state_machine.vi"("State(s) in Front (\"\")"=w261, "State(s) in (\"\")"=w265) -> ("States Out"=w264:string)  [unwired: 13 in]
          }
          frame "Macro: Exit" {
            # "Exit Macro\n(This is called once, when the VI exits)"
            n84 = Unbundle By Name(w272) -> ("Core.Close Panel on Exit?"=w271:bool)
            n85 = Select(t="UI: Front Panel State >> Close", s=w271, f="") -> (s? t:f=w268:string)
            n86 = call <vilib>:"Add State(s) to Queue__jki_lib_state_machine.vi"("State(s) in (\"\")"=w268, "State(s) at Back (\"\")"="Remote: Disconnect\nData: Cleanup\nExit") -> ("States Out"=w266:string)  [unwired: 13 in]
            n87 = call <vilib>:"Add State(s) to Queue__jki_lib_state_machine.vi"("State(s) in Front (\"\")"=w266, "State(s) in (\"\")"=w275) -> ("States Out"=w274:string)  [unwired: 13 in]
          }
          frame "---------- Remote ----------" {
            # "Template Separator\n(You can make a copy of, or modify, this frame)"
            n88 = Unbundle By Name(w282) -> ("RemoteControl"=w285:refnum<class "RemoteControl.lvclass">)
            n89 = call <userlib>:"Send and Receive.vi"("timeout (ms) [500]"=500, "error in (no error)"=w281, "RemoteControl in"=w285) -> ("error out"=w278:errorcluster, "Data out"=w277:variant, "Command out"=w276:string, "RemoteControl out"=w284:refnum<class "RemoteControl.lvclass">)  [unwired: 5 in]
            n90 = call "JSON to LVtype.vim"("type"="", "error in (no error)"=w278, "JSON Data in"=w277, 10:w276) -> ()  [unwired: 6 in, 2 out]
            n91 = Bundle By Name(cluster=w282, "RemoteControl"=w284) -> (w283:T9)
            n92 = call <vilib>:"Add State(s) to Queue__jki_lib_state_machine.vi"("State(s) in (\"\")"=w287) -> ("States Out"=w286:string)  [unwired: 14 in]
          }
          frame "Remote: Connect" {
            # "Template Separator\n(You can make a copy of, or modify, this frame)"
            n93 = Unbundle By Name(w302) -> ("RemoteControl"=w301:refnum<class "RemoteControl.lvclass">, "IV Settings.Port"=w298:u32)
            n94 = call <userlib>:"Connect.vi"(6:RC_Com_Type--enum."ZMQ" ("RC Type"), "error in (no error)"=w300, "Port"=w298, "address"="", "RemoteControl in"=w301) -> ("error out"=w290:errorcluster, "RemoteControl out"=w292:refnum<class "RemoteControl.lvclass">)  [unwired: 5 in]
            n95 = call <userlib>:"Send and Receive.vi"("timeout (ms) [500]"=500, "error in (no error)"=w290, "Command"="ACK", "RemoteControl in"=w292) -> ("error out"=w289:errorcluster, "RemoteControl out"=w291:refnum<class "RemoteControl.lvclass">)  [unwired: 4 in, 2 out]
            n96 = Select(t=0, s=w289, f=1) -> (s? t:f=w296:i32)
            n97 = Bundle By Name(cluster=w302, "RemoteControl"=w291, "Plugin Status"=w296) -> (w303:T9)
            n98 = call <vilib>:"Add State(s) to Queue__jki_lib_state_machine.vi"("State(s) in (\"\")"=w305) -> ("States Out"=w304:string)  [unwired: 14 in]
          }
          frame "Remote: Disconnect" {
            # "Template Separator\n(You can make a copy of, or modify, this frame)"
            n99 = Unbundle By Name(w313) -> ("RemoteControl"=w312:refnum<class "RemoteControl.lvclass">, "Plugin Status"=w309:i32)
            n100 = call <userlib>:"Disconnect.vi"("error in (no error)"=w310, "RemoteControl in"=w312) -> ("error out"=w306:errorcluster, "RemoteControl out"=w311:refnum<class "RemoteControl.lvclass">)  [unwired: 8 in]
            n101 = Select(t=w309, s=w306, f=2) -> (s? t:f=w307:i32)
            n102 = Bundle By Name(cluster=w313, "RemoteControl"=w311, "Plugin Status"=w307) -> (w314:T9)
            n103 = call <vilib>:"Add State(s) to Queue__jki_lib_state_machine.vi"("State(s) in (\"\")"=w316) -> ("States Out"=w315:string)  [unwired: 14 in]
          }
          frame "Remote: IV_STATUS" {
            # "Template Separator\n(You can make a copy of, or modify, this frame)"
            n104 = Unbundle By Name(w328) -> ("RemoteControl"=w331:refnum<class "RemoteControl.lvclass">, "Status"=w322:enum16{"IDLE", "RUNNING", "FINISHED", "ABORTED"})
            n105 = call <userlib>:"Send and Receive.vi"("timeout (ms) [500]"=1000, "error in (no error)"=w318, "Command"="IV_STATUS", "RemoteControl in"=w331) -> ("error out"=w326:errorcluster, "Data out"=w325:variant, "RemoteControl out"=w330:refnum<class "RemoteControl.lvclass">)  [unwired: 4 in, 1 out]
            n106 = call "JSON to LVtype.vim"("type"="", "error in (no error)"=w326, "JSON Data in"=w325) -> ("error out"=w321:errorcluster, "Data out"=w323:string)  [unwired: 7 in]
            n107 = Scan From String(input string=w323, error in=w321, default 1=w322) -> (error out=w319:errorcluster, output 1=w320:enum16{"IDLE", "RUNNING", "FINISHED", "ABORTED"})  [unwired: 2 in, 2 out]
            n108 = Bundle By Name(cluster=w328, "RemoteControl"=w330, "Status"=w320) -> (w329:T9)
            n109 = call <vilib>:"Add State(s) to Queue__jki_lib_state_machine.vi"("State(s) in (\"\")"=w333) -> ("States Out"=w332:string)  [unwired: 14 in]
          }
          frame "Remote: IV_RUN" {
            # "If you try to put this straight in the names will be IV Settings.Time"
            # "#todo\nMake the interface consistent all the way around"
            # "Template Separator\n(You can make a copy of, or modify, this frame)"
            n110 = Unbundle By Name(w360) -> ("Plugin Status"=w344:i32, "Status"=w349:enum16{"IDLE", "RUNNING", "FINISHED", "ABORTED"}, "RemoteControl"=w363:refnum<class "RemoteControl.lvclass">, "IV Settings.Pattern"=w355:T7, "IV Settings.Cycles"=w356:i32, "IV Settings.Rate"=w357:dbl, "IV Settings.End"=w354:dbl, "IV Settings.Start"=w353:dbl, "IV Settings.Time"=w343:dbl, "IV Settings.Points"=w342:dbl[])  [unwired: 1 out]
            n111 = Bundle By Name(cluster=T6 {"Pattern"=enum."Ramp /", "Cycles"=0, "Rate"=0.0, "End"=0.0, "Start"=0.0}, "Pattern"=w355, "Cycles"=w356, "Rate"=w357, "End"=w354, "Start"=w353) -> ()  [unwired: 1 out]
            n112 = Bundle By Name(cluster=cluster{"Time":dbl, "Points":dbl[]} {"Time"=1.0, "Points"=[0.0, 1.0]} ("input cluster"), "Time"=w343, "Points"=w342) -> (w336:cluster{"Time":dbl, "Points":dbl[]})
            n113 = call <userlib>:"Send and Receive.vi"("timeout (ms) [500]"=2000, "error in (no error)"=w338, "Data"=w336, "Command"="IV_RUN", "RemoteControl in"=w363) -> ("error out"=w339:errorcluster, "Data out"=w350:variant, "Command out"=w335:string, "RemoteControl out"=w362:refnum<class "RemoteControl.lvclass">)  [unwired: 3 in]
            n114 = call "JSON to LVtype.vim"("type"="", "error in (no error)"=w339, "JSON Data in"=w350, 10:w335) -> ("error out"=w351:errorcluster, "Data out"=w334:string)  [unwired: 6 in]
            n115 = call "Debug Write.vim"("prefix (\"\")"="This is the return from the plugin: " ("prefix (\"\")"), "error in (no error)"=w339, "value"=w334) -> ()  [unwired: 8 in, 1 out]
            n116 = Scan From String(input string=w334, error in=w351, default 1=w349) -> (error out=w347:errorcluster, output 1=w348:enum16{"IDLE", "RUNNING", "FINISHED", "ABORTED"})  [unwired: 2 in, 2 out]
            n117 = Select(t=w344, s=w339, f=3 ("Plugin Status")) -> (s? t:f=w346:i32)
            n118 = Bundle By Name(cluster=w360, "RemoteControl"=w362, "Status"=w348, "Plugin Status"=w346) -> (w361:T9)
            n119 = call <vilib>:"Add State(s) to Queue__jki_lib_state_machine.vi"("State(s) in (\"\")"=w365) -> ("States Out"=w364:string)  [unwired: 14 in]
          }
          frame "Remote: IV_ABORT" {
            # "Template Separator\n(You can make a copy of, or modify, this frame)"
            n120 = Unbundle By Name(w379) -> ("RemoteControl"=w382:refnum<class "RemoteControl.lvclass">, "Status"=w370:enum16{"IDLE", "RUNNING", "FINISHED", "ABORTED"})
            n121 = call <userlib>:"Send and Receive.vi"("timeout (ms) [500]"=500, "error in (no error)"=w366, "Command"="IV_ABORT", "RemoteControl in"=w382) -> ("error out"=w374:errorcluster, "Data out"=w376:variant, "Command out"=w375:string, "RemoteControl out"=w381:refnum<class "RemoteControl.lvclass">)  [unwired: 4 in]
            n122 = call "JSON to LVtype.vim"("type"="", "error in (no error)"=w374, "JSON Data in"=w376, 10:w375) -> ("error out"=w372:errorcluster, "Data out"=w373:string)  [unwired: 6 in]
            n123 = Scan From String(input string=w373, error in=w372, default 1=w370) -> (error out=w371:errorcluster, output 1=w369:enum16{"IDLE", "RUNNING", "FINISHED", "ABORTED"})  [unwired: 2 in, 2 out]
            n124 = Bundle By Name(cluster=w379, "RemoteControl"=w381, "Status"=w369, "Plugin Status"=5) -> (w380:T9)
            n125 = call <vilib>:"Add State(s) to Queue__jki_lib_state_machine.vi"("State(s) in (\"\")"=w384) -> ("States Out"=w383:string)  [unwired: 14 in]
          }
          frame "---------- Timeout ----------" {
            # "Do not put any code in this frame.\n(It is a separator no-op. You can make a copy of this frame to create a new Macro frame)"
            n126 = call <vilib>:"Add State(s) to Queue__jki_lib_state_machine.vi"("State(s) in (\"\")"=w388) -> ("States Out"=w387:string)  [unwired: 14 in]
          }
          frame "Timeout: Abort" {
            # "Do not put any code in this frame.\n(It is a separator no-op. You can make a copy of this frame to create a new Macro frame)"
            n127 = Unbundle By Name(w395) -> ("Pattern Data.Name"=w394:string)
            n128 = Concatenate Strings("Object " ("Message"), w394, " Timed Out!!" ("string")) -> (w392:string)
            n129 = call "Display Message to User"("error in (no error)"=w390, "Message"=w392) -> ("error out"=w391:errorcluster)  [unwired: 8 in, 1 out]
            n130 = call <vilib>:"Add State(s) to Queue__jki_lib_state_machine.vi"("State(s) in Front (\"\")"="Macro: Abort", "State(s) in (\"\")"=w398) -> ("States Out"=w397:string)  [unwired: 13 in]
          }
          frame "Timeout: Check" {
            # "Do not put any code in this frame.\n(It is a separator no-op. You can make a copy of this frame to create a new Macro frame)"
            n131 = Unbundle By Name(w405) -> ("Timeout"=w403:u32)
            n132 = Tick Count (ms)() -> (millisecond timer value=w404:u32)
            n133 = Greater?(x=w404, y=w403) -> (0:w402:bool)
            n134 = Select(t="Timeout: Abort", s=w402, f="") -> (s? t:f=w399:string)
            n135 = call <vilib>:"Add State(s) to Queue__jki_lib_state_machine.vi"("State(s) in Front (\"\")"=w399, "State(s) in (\"\")"=w408) -> ("States Out"=w407:string)  [unwired: 13 in]
          }
          frame "Timeout: Calculate" {
            # "Do not put any code in this frame.\n(It is a separator no-op. You can make a copy of this frame to create a new Macro frame)"
            n136 = disable-structure shown="Enabled" {
              disable-tunnel: w410 -> [w421 w450]
              disable-tunnel: [w420 w443] -> w409
              frame Disabled {
                # "Divide by rate of ramp"
                # "Total number of volts to ramp across"
                # "Ramps up and back down are twice the time"
                # "Add 10 seconds per cycle"
                n137 = Unbundle By Name(w421) -> ("IV Settings.Pattern"=w437:T7, "IV Settings.Rate"=w440:dbl, "IV Settings.End"=w442:dbl, "IV Settings.Start"=w441:dbl, "IV Settings.Cycles"=w417:i32)
                n138 = Subtract(x=w442, y=w441) -> (x-y=w439:dbl)
                n139 = Divide(x=w439, y=w440) -> (x/y=w438:dbl)
                n140 = Absolute Value(x=w438) -> (abs(x)=w428:dbl)
                n141 = Equal?(x=T7."Smooth Ramp _/\\_" ("IV Settings.Pattern"), y=w437) -> (x = y?=w434:bool)
                n142 = Equal?(x=w437, y=T7."Ramp /\\" ("IV Settings.Pattern")) -> (x = y?=w433:bool)
                n143 = Or(x=w434, y=w433) -> (x .or. y?=w432:bool)
                n144 = Select(t=2.0, s=w432, f=1.0) -> (s? t:f=w431:dbl)
                n145 = Multiply(x=w431, y=w428) -> (x*y=w419:dbl)
                n146 = Multiply(x=w419, y=w417) -> (x*y=w418:dbl)
                n147 = Multiply(x=w417, y=10) -> (x*y=w415:i32)
                n148 = Add(x=w418, y=w415) -> (x+y=w427:dbl)
                n149 = Add(x=w427, y=10.0) -> (x+y=w425:dbl)
                n150 = Tick Count (ms)() -> (millisecond timer value=w422:u32)
                n151 = Multiply(x=w425, y=1000.0) -> (x*y=w423:dbl)
                n152 = Add(x=w423, y=w422) -> (x+y=w420:dbl)
              }
              frame Enabled {
                n153 = Unbundle By Name(w450) -> ("IV Settings.Time"=w449:dbl)
                n154 = Add(x=w449, y=30.0) -> (x+y=w447:dbl)
                n155 = Multiply(x=w447, y=1000.0) -> (x*y=w445:dbl)
                n156 = Tick Count (ms)() -> (millisecond timer value=w444:u32)
                n157 = Add(x=w445, y=w444) -> (x+y=w443:dbl)
              }
            }
            n158 = Bundle By Name(cluster=w410, "Timeout"=w409) -> (w411:T9)
            n159 = call <vilib>:"Add State(s) to Queue__jki_lib_state_machine.vi"("State(s) in (\"\")"=w414) -> ("States Out"=w413:string)  [unwired: 14 in]
          }
        }
      }
      n160 = Unbundle By Name(w12) -> ("Application"=w15:refnum<k7>)
    }
    frame True {
      # "Aborted. Do not run the plugin."
    }
  }
  "error out" <- w11
  "Application Out" <- w5
